vi "Update_all.vi"(7 "# axis":i32, 8 "error in (no error)":errorcluster, 11 "VISA resource name":refnum<visa-resource-name>) -> (0 "error out":errorcluster, 1 "Moving":bool, 2 "Currrent postion":dbl[](array[numeric]), 3 "tickcount_pos":u32, 5 "MotorDisabled":bool)   [LabVIEW 2012, in "Micos_uic.lvlib"]
doc: "Performs an instrument error query before terminating the software connection to the instrument."
uses:
  Micos_uic.lvlib
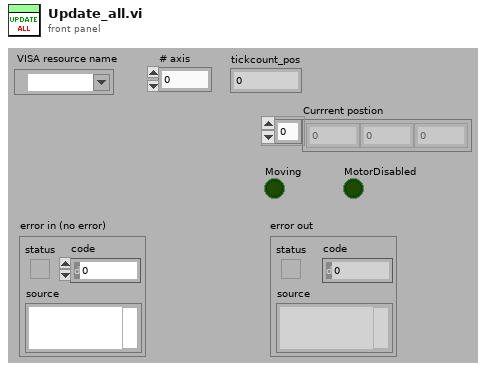
[diagram p1: front panel]
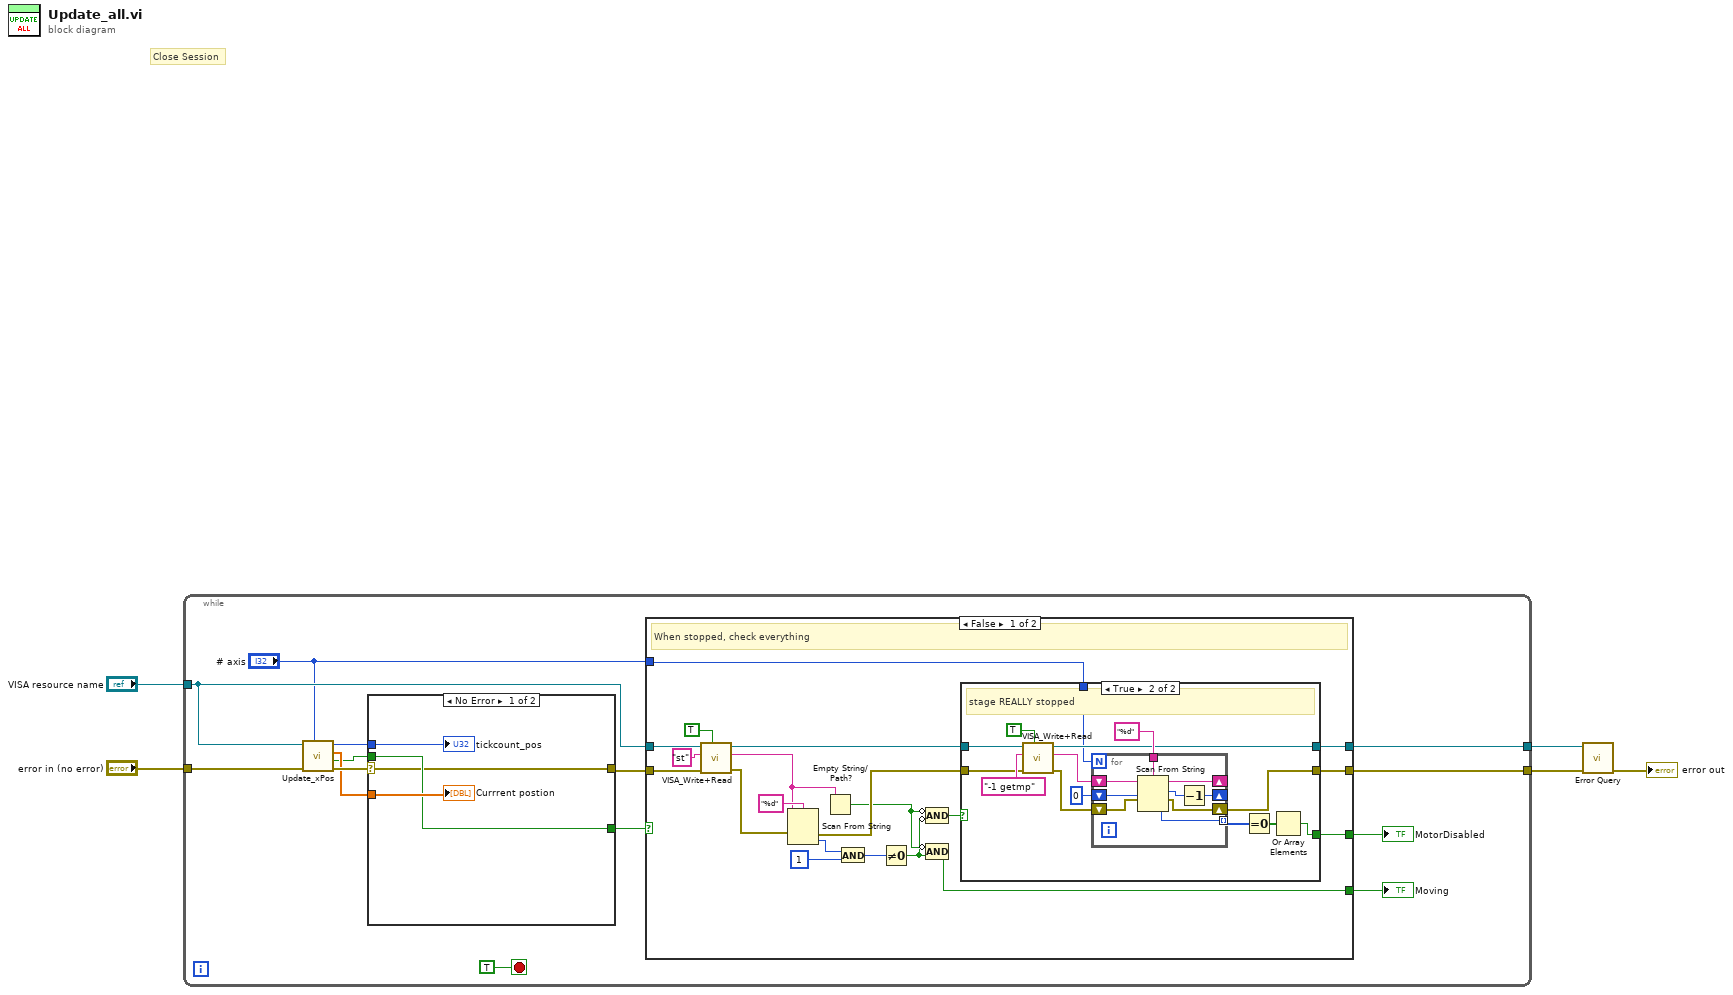
[diagram p0: block diagram]
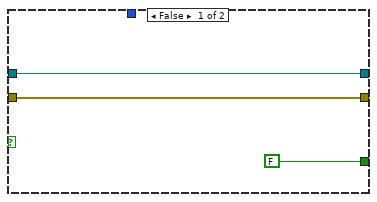
[diagram p2: hidden frame]
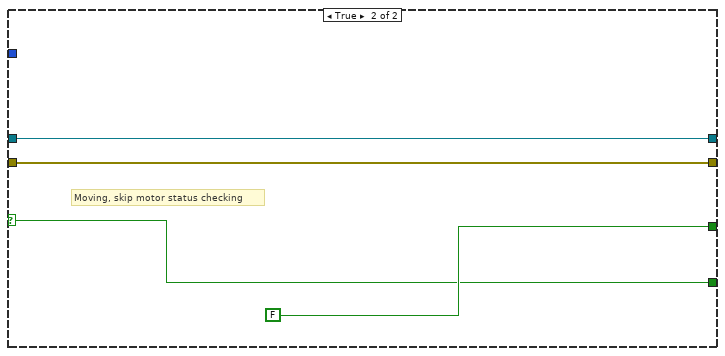
[diagram p3: hidden frame]
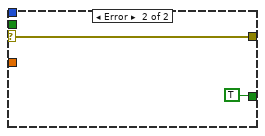
[diagram p4: hidden frame]
diagram:
  # "Close Session"
  n1 = while {
    tunnel: "error in (no error)" -> [w11]
    tunnel: "VISA resource name" -> [w13]
    tunnel: [w15] -> w1
    tunnel: [w14] -> w2
    stop <- TRUE stop-if-true
    n2 = call "Update_xPos.vi"("NumOfAxis"="# axis", "error in (no error)"=w11, "VISA resource name"=w13) -> ("error out"=w10:errorcluster, "x_Moving"=w7:bool, "Position"=w8:dbl[], "tickcount_pos"=w9:u32)  [unwired: 5 in]
    n3 = case shown="No Error" w10 {
      selector: w10 -> [w70 w75]
      tunnel: w9 -> [w73 _]
      tunnel: w8 -> [w72 _]
      tunnel: [w70 w75] -> w16
      tunnel: w7 -> [w71 _]
      tunnel: [w71 TRUE] -> w18
      frame No Error {
        "Currrent postion" <- w72
        "tickcount_pos" <- w73
      }
      frame Error {
      }
    }
    n4 = case shown="False" w18 {
      selector: w18 -> [_ w66]
      tunnel: [w21 FALSE] -> w17
      tunnel: w13 -> [w29 w68]
      tunnel: "# axis" -> [w20 _]
      tunnel: [w27 w68] -> w15
      tunnel: [w26 w67] -> w14
      tunnel: w16 -> [w33 w67]
      tunnel: [w32 w66] -> w6
      frame False {
        # "When stopped, check everything"
        n5 = call "VISA_Write+Read.vi"("Read?"=TRUE, "error in (no error)"=w33, "Write Buffer"="st" ("string"), "VISA resource name"=w29) -> ("error out"=w37:errorcluster, "readout"=w34:string, "VISA resource name out"=w28:refnum<visa-resource-name>)  [unwired: 5 in]
        n6 = Scan From String(format string="%d", input string=w34, error in=w37) -> (error out=w25:errorcluster, output 1=w31:i32)  [unwired: 2 in, 2 out]
        n7 = Empty String/Path?(string/path=w34) -> (empty?=w24:bool)
        n8 = And(x=w31, y=1) -> (x .and. y?=w35:i32)
        n9 = Not Equal To 0?(x=w35) -> (x != 0?=w23:bool)
        n10 = Compound Arithmetic op=AND(invert w24, invert w23) -> (w22:bool)
        n11 = Compound Arithmetic op=AND(invert w24, w23) -> (w32:bool)
        n12 = case shown="True" w22 {
          tunnel: w28 -> [w41 w51]
          tunnel: [w41 w50] -> w27
          tunnel: [w42 w49] -> w26
          tunnel: w25 -> [w42 w48]
          tunnel: [FALSE w45] -> w21
          tunnel: w20 -> [_ w44]
          frame False {
          }
          frame True {
            # "stage REALLY stopped"
            n13 = call "VISA_Write+Read.vi"("Read?"=TRUE, "error in (no error)"=w48, "Write Buffer"="-1 getmp" ("string"), "VISA resource name"=w51) -> ("error out"=w54:errorcluster, "readout"=w55:string, "VISA resource name out"=w50:refnum<visa-resource-name>)  [unwired: 5 in]
            n14 = for {
              N: w44 -> [_]
              tunnel: "%d" ("format string") -> [w63]
              shift-right: [w62] -> w49
              shift-left: w54 -> [w64]
              shift-right: [w61] -> _
              shift-left: w55 -> [w65]
              shift-right: [w57] -> _
              shift-left: u32 0 -> [w59]
              tunnel: [w58] -> w47 mode=indexing
              n15 = Scan From String(format string=w63, input string=w65, initial scan location=w59, error in=w64) -> (remaining string=w61:string, offset past scan=w60:u32, error out=w62:errorcluster, output 1=w58:i32)  [unwired: 1 in]
              n16 = Decrement(x=w60) -> (x-1=w57:u32)
            }
            n17 = Equal To 0?(x=w47) -> (x = 0?=w46:bool[])
            n18 = Or Array Elements(Boolean array=w46) -> (logical OR=w45:bool)
          }
        }
      }
      frame True {
        # "Moving, skip motor status checking"
      }
    }
    "MotorDisabled" <- w17
    "Moving" <- w6
  }
  n19 = call "Error Query.vi"("error in (no error)"=w2, "VISA resource name"=w1) -> ("error out"=→"error out":errorcluster)  [unwired: 6 in, 3 out]
